vi "ModelCheckCell.vi"(9 "checkpars":i32, 10 "COMPNTSN_in":string, 11 "ModelCheckArray":string[](array[string])) -> (1 "COMPNTID":string, 2 "COMPNTSN":string, 3 "OK?":bool)   [LabVIEW 2014]
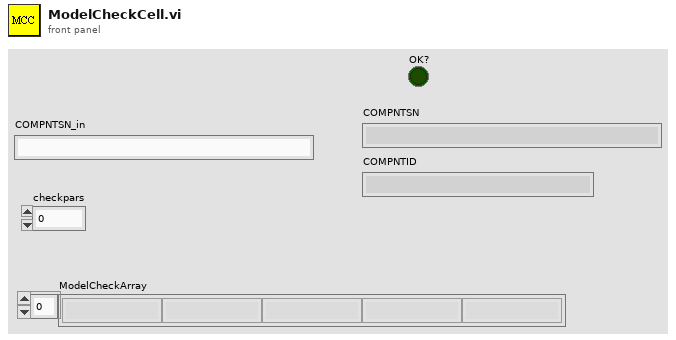
[diagram p1: front panel]
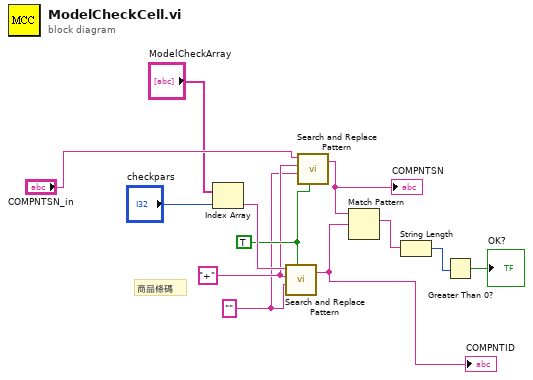
[diagram p0: block diagram]
diagram:
  w8 = TRUE ("replace all? (F)")
  w6 = "" ("replace string (\"\")")
  w7 = "+" ("regular expression (\"\")")
  # "商品條碼"
  n1 = Index Array(array="ModelCheckArray", index="checkpars") -> (element=w10:string)
  n2 = call <vilib>:"Search and Replace Pattern.vi"("string"=w10, "regular expression (\"\")"=w7, "replace string (\"\")"=w6, "replace all? (F)"=w8) -> ("result string"=w5:string)  [unwired: 1 in, 1 out]
  "COMPNTID" <- w5
  n3 = call <vilib>:"Search and Replace Pattern.vi"("string"="COMPNTSN_in", "regular expression (\"\")"=w7, "replace string (\"\")"=w6, "replace all? (F)"=w8) -> ("result string"=w9:string)  [unwired: 1 in, 1 out]
  "COMPNTSN" <- w9
  n4 = Match Pattern(string=w9, regular expression=w5) -> (match substring=w12:string)  [unwired: 1 in, 3 out]
  n5 = String Length(string=w12) -> (length=w11:i32)
  n6 = Greater Than 0?(x=w11) -> (x > 0?=→"OK?":bool)
